vi "PDCConvertTrigg.vi"(10 "TriggerValue":u16, 11 "TriggerStrings":string[](array[string])) -> (3 "TriggerMode":u32)   [LabVIEW 2015]
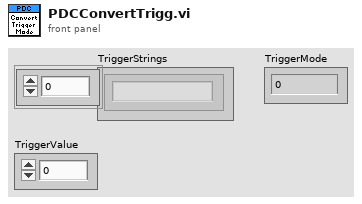
[diagram p1: front panel]
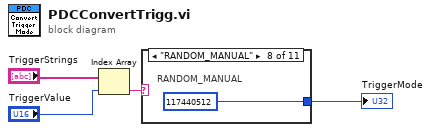
[diagram p0: block diagram]
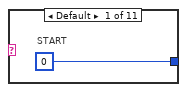
[diagram p2: hidden frame]
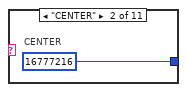
[diagram p3: hidden frame]
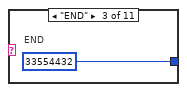
[diagram p4: hidden frame]
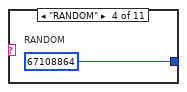
[diagram p5: hidden frame]
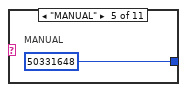
[diagram p6: hidden frame]
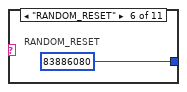
[diagram p7: hidden frame]
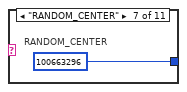
[diagram p8: hidden frame]
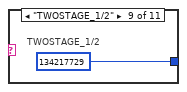
[diagram p9: hidden frame]
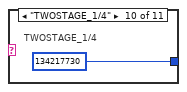
[diagram p10: hidden frame]
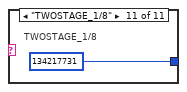
[diagram p11: hidden frame]
diagram:
  n1 = Index Array(array="TriggerStrings", index="TriggerValue") -> (element=w3:string)
  n2 = case shown="\"RANDOM_MANUAL\"" w3 {
    tunnel: [u32 0 ("nMode") u32 16777216 ("nMode") u32 33554432 ("nMode") u32 67108864 ("nMode") u32 50331648 ("nMode") u32 83886080 ("nMode") u32 100663296 ("nMode") u32 117440512 ("nMode") u32 134217729 ("nMode") u32 134217730 ("nMode") u32 134217731 ("nMode")] -> w4
    frame Default {
      # "START"
    }
    frame "CENTER" {
      # "CENTER"
    }
    frame "END" {
      # "END"
    }
    frame "RANDOM" {
      # "RANDOM"
    }
    frame "MANUAL" {
      # "MANUAL"
    }
    frame "RANDOM_RESET" {
      # "RANDOM_RESET"
    }
    frame "RANDOM_CENTER" {
      # "RANDOM_CENTER"
    }
    frame "RANDOM_MANUAL" {
      # "RANDOM_MANUAL"
    }
    frame "TWOSTAGE_1/2" {
      # "TWOSTAGE_1/2"
    }
    frame "TWOSTAGE_1/4" {
      # "TWOSTAGE_1/4"
    }
    frame "TWOSTAGE_1/8" {
      # "TWOSTAGE_1/8"
    }
  }
  "TriggerMode" <- w4
